vi "get_IDs.vi"() -> (0 "error out 3":errorcluster, 1 "CmdLib Out":refnum<k24>, 2 "DeviceKey List Out":string[](array[string]), 3 "Identification List":string[](array[string]), 4 "IDs":i32[](array[numeric]), 5 "Device Key":string[](array[string]))   [LabVIEW 2014]
uses:
  C:/Program Files/New Focus/New Focus Picomotor Application/Samples/CmdLib.dll
  Program Files/New Focus/New Focus Picomotor Application/Samples/CmdLib.dll
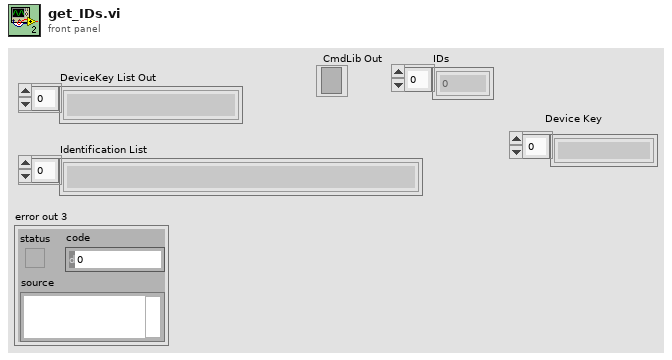
[diagram p1: front panel]
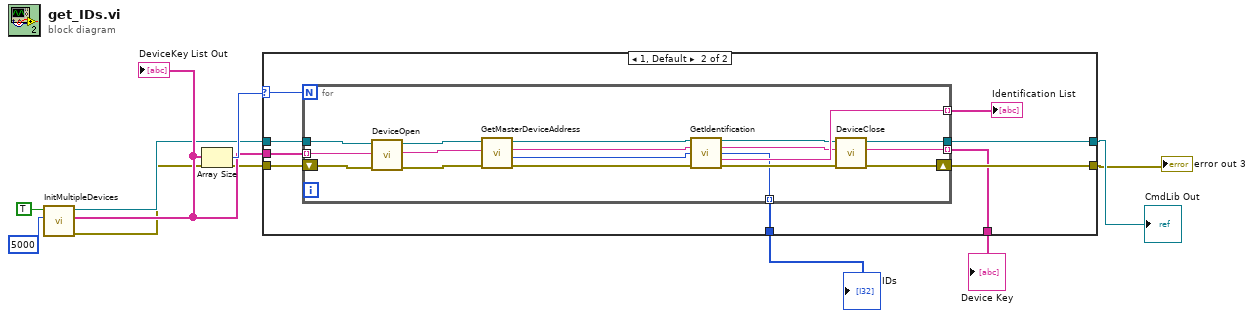
[diagram p0: block diagram]
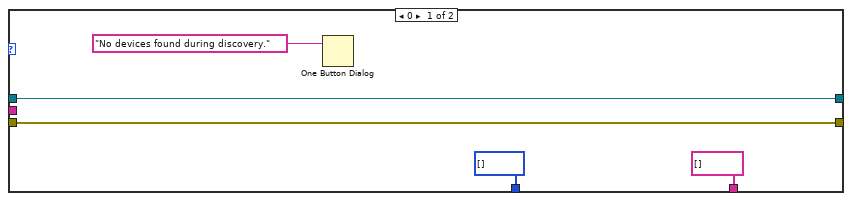
[diagram p2: hidden frame]
diagram:
  n1 = call "InitMultipleDevices.vi"("msecDelayForDiscovery"=5000, "logging"=TRUE) -> ("error out"=w5:errorcluster, "DeviceKey List Out"=w7:string[], "CmdLib Out"=w6:refnum<k24>)  [unwired: 3 in]
  "DeviceKey List Out" <- w7
  n2 = Array Size(array=w7) -> (size(s)=w8:i32)
  n3 = case shown="1, Default" w8 {
    selector: w8 -> [_ w24]
    tunnel: w7 -> [_ w23]
    tunnel: w6 -> [w14 w22]
    tunnel: w5 -> [w15 w21]
    tunnel: [w15 w20] -> w3
    tunnel: [w14 w19] -> w4
    tunnel: [i32[] [] w17] -> w2
    tunnel: [string[] [] w16] -> w1
    frame 0 {
      n4 = One Button Dialog(message="No devices found during discovery.") -> ()  [unwired: 1 in, 1 out]
    }
    frame 1, Default {
      n5 = for {
        N: w24 -> [_]
        tunnel: w23 -> [w38] mode=indexing
        tunnel: [w42] -> w18 mode=indexing
        tunnel: w22 -> [w41]
        tunnel: [w40] -> w19
        shift-right: [w36] -> w20
        shift-left: w21 -> [w37]
        tunnel: [w26] -> w17 mode=indexing
        tunnel: [w25] -> w16 mode=indexing
        n6 = call "DeviceOpen.vi"("error in (no error)"=w37, "DeviceKey In"=w38, "CmdLib In"=w41) -> ("error out"=w31:errorcluster, "DeviceKey Out"=w32:string, "CmdLib Out"=w33:refnum<k24>)  [unwired: 2 in]
        n7 = call "GetMasterDeviceAddress.vi"("error in (no error)"=w31, "DeviceKey In"=w32, "CmdLib In"=w33) -> ("error out"=w27:errorcluster, "Device Address"=w30:i32, "DeviceKey Out"=w29:string, "CmdLib Out"=w28:refnum<k24>)  [unwired: 1 in]
        n8 = call "GetIdentification.vi"("CmdLib In"=w28, "DeviceKey In"=w29, "Device Address In"=w30, "error in (no error)"=w27) -> ("CmdLib Out"=w39:refnum<k24>, "DeviceKey Out"=w34:string, "Device Address Out"=w26:i32, "Identification"=w42:string, "error out"=w35:errorcluster)  [unwired: 7 in]
        n9 = call "DeviceClose.vi"("error in (no error)"=w35, "DeviceKey In"=w34, "CmdLib In"=w39) -> ("error out"=w36:errorcluster, "DeviceKey Out"=w25:string, "CmdLib Out"=w40:refnum<k24>)  [unwired: 2 in]
      }
      "Identification List" <- w18
    }
  }
  "error out 3" <- w3
  "CmdLib Out" <- w4
  "IDs" <- w2
  "Device Key" <- w1
